vi "Read Current project context.vi"(9 "Current ProjectItem":refnum<class "ProjectItem.lvclass">, 11 "BuildManager in":refnum<class "BuildManager.lvclass">) -> (1 "Project context":refnum<vi>, 3 "BuildManager out":refnum<class "BuildManager.lvclass">)   [LabVIEW 2019, in "SolutionBuilder.lvlib" / "BuildManager.lvclass"]
uses:
  BuildManager.lvclass
  BuildManager.lvclass/BuildManager.ctl
  ProjectItem/ProjectItem.lvclass
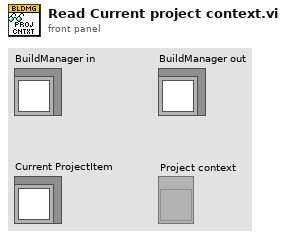
[diagram p1: front panel]
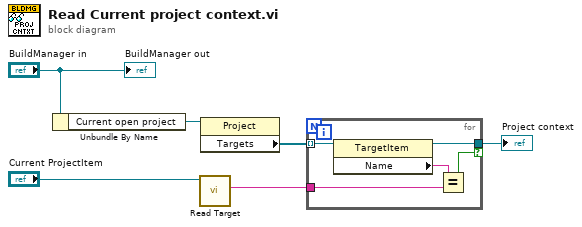
[diagram p0: block diagram]
diagram:
  n1 = Unbundle By Name("BuildManager in") -> ("Current open project"=w4:refnum<vi>)
  n2 = call "Read Target.vi"("ProjectItem in"="Current ProjectItem") -> ("Target"=w1:string)  [unwired: 9 in, 1 out]
  n3 = property class="Project"(reference=w4) -> ("Targets"=w5:refnum<vi>[])  [unwired: 1 in, 2 out]
  n4 = for {
    tunnel: w5 -> [w11] mode=indexing
    tunnel: w1 -> [w9]
    tunnel: [w8] -> w3 if=w7
    n5 = property class="TargetItem"(reference=w11) -> (reference out=w8:refnum<vi>, "Name"=w10:string)  [unwired: 1 in, 1 out]
    n6 = Equal?(x=w10, y=w9) -> (x = y?=w7:bool)
  }
  "Project context" <- w3
  "BuildManager out" <- "BuildManager in"
